vi "Switch Heater Current (Set).vi"(6 "ISOBUS address":T4=-1 caption="ISOBUS address (-1)", 8 "error in":errorcluster, 9 "Unit":T1, 10 "Swh Htr Current":dbl caption="Switch Heater Current (mA)" min=0.0 max=125.0 step=0.01 format="%#.2f", 11 "Mercury Reference In":T5) -> (0 "error out":errorcluster, 2 "Response":T2, 3 "Mercury Reference Out":T5, 4 "Valid?":T3)   [LabVIEW 2016, in "Mercury iXX.lvlib" / "Magnet.lvlib"]
doc: "Set the current configuration for the Switch Heater Current (mA).\n\nNB: The instrument must be in Engineering mode to set this item."
uses:
  Magnet.lvlib
  Controls/Mercury Reference.ctl
  Controls/Comms Transport Layer.ctl
  Private/Controls/Query Dynamic Reference.ctl
  Controls/ISOBus Address.ctl
  Controls/Is Valid LED.ctl
  Controls/Response String.ctl
  Controls/Unit String.ctl
  Private/Controls/Command Verbs.ctl
  Mercury iXX.lvlib
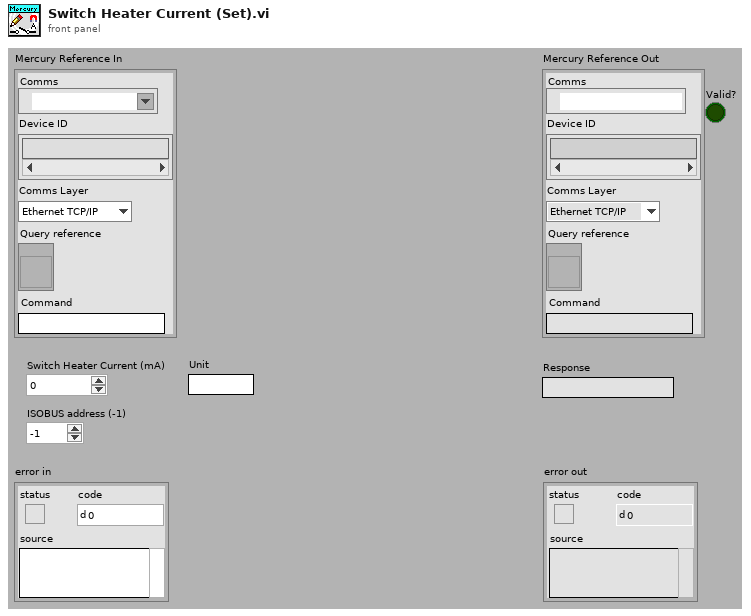
[diagram p1: front panel]
types:
  T1 = typedef "Mercury iXX.lvlib/Unit String.ctl" = string
  T2 = typedef "Mercury iXX.lvlib/Response String.ctl" = string
  T3 = typedef "Mercury iXX.lvlib/Is Valid LED.ctl" = bool
  T4 = typedef "Mercury iXX.lvlib/ISOBus Address.ctl" = i32
  T5 = typedef "Mercury iXX.lvlib/Mercury Reference.ctl" = cluster{"Comms":refnum<visa-resource-name>, "Device ID":string[], "Comms Layer":T6, "Command":string, "Query reference":T7}
  T6 = typedef "Mercury iXX.lvlib/Comms Transport Layer.ctl" = enum16{"Ethernet TCP/IP", "USB", "ISOBus - RS-232", "GPIB"}
  T7 = typedef "Mercury iXX.lvlib/Query Dynamic Reference.ctl" = refnum<vi>
  T8 = typedef "Mercury iXX.lvlib/Command Verbs.ctl" = string
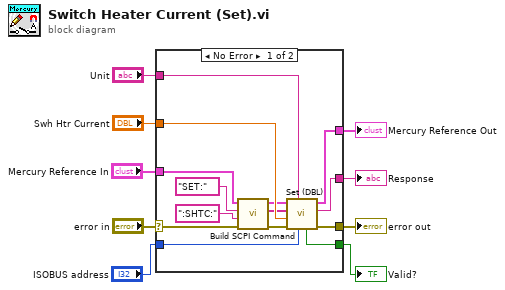
[diagram p0: block diagram]
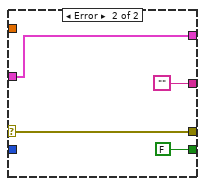
[diagram p2: hidden frame]
diagram:
  n1 = case shown="No Error" "error in" {
    selector: "error in" -> [w15 w27]
    tunnel: "Mercury Reference In" -> [w16 w26]
    tunnel: "ISOBUS address" -> [w23 _]
    tunnel: [w22 T3 FALSE ("Valid?")] -> w7
    tunnel: [w21 w27] -> w6
    tunnel: [w20 ""] -> w5
    tunnel: [w19 w26] -> w4
    tunnel: "Swh Htr Current" -> [w18 _]
    tunnel: "Unit" -> [w10 _]
    frame No Error {
      n2 = call "Build SCPI Command.vi"("error in"=w15, "Noun(s)"=":SHTC:" ("Command"), "Verb"=T8 "SET:", "Mercury Reference In"=w16) -> ("error out"=w11:errorcluster, "SCPI Message(s)"=w17:string[], "Mercury Reference Out"=w12:T5)  [unwired: 5 out]
      n3 = call "Set (DBL).vi"("ISOBUS address"=w23, "Unit"=w10, "error in"=w11, "Command Value (Dbl)"=w18, "SCPI Message(s)"=w17, "Mercury Reference In"=w12) -> ("error out"=w21:errorcluster, "Response"=w20:T2, "Mercury Reference Out"=w19:T5, "Valid?"=w22:T3)  [unwired: 2 out]
    }
    frame Error {
    }
  }
  "Mercury Reference Out" <- w4
  "error out" <- w6
  "Valid?" <- w7
  "Response" <- w5
